vi "NI VeriStand - Start Single Waveform (CDB).vi"(8 "error in (no error)":errorcluster, 10 "t0":timestamp, 11 "Single Waveform Write Session (CDB) in":refnum<class "Single Waveform Write (CDB).lvclass">) -> (0 "error out":errorcluster, 3 "Single Waveform Write Session (CDB) out":refnum<class "Single Waveform Write (CDB).lvclass">)   [LabVIEW 2020, in "NI_VS Custom Device Waveform API.lvlib" / "Single Waveform Write (CDB).lvclass"]
doc: "Sets the start time (t0) for the waveform data you want to write with the Write Waveform(s) VI. NI VeriStand considers all data the custom device writes to a waveform be continuous unless this VI executes again with a different start time."
uses:
  Single Waveform Write (CDB).lvclass
  D:/p4/penguin/lvaddon/Veristand/master/src/LabVIEW/vilib/NI VeriStand/Custom Device Waveform API/Waveform Session.lvclass
  Waveform Session.lvclass/Waveform Session.ctl
  Single Waveform Write (CDB).lvclass/Single Waveform Write (CDB).ctl
  Internal Comm Classes/WPL Comm/WPL Comm.lvclass/WPL Comm.ctl
  Internal Comm Classes/WPL Comm/Set t0 on Variant.vi
  Internal Comm Classes/WPL Comm/Send WPL Command.vi
  Internal Comm Classes/WPL Comm/Convert Q Error to Shutdown Error.vi
  Internal Comm Classes/WPL Comm/WPL Comm (1D CDB)/WPL Comm (1D CDB).lvclass
  D:/p4/penguin/lvaddon/Veristand/master/src/LabVIEW/vilib/NI VeriStand/Custom Device Waveform API/Internal Comm Classes/WPL Comm/WPL Comm.lvclass
  <vilib>/Utility/error.llb/Error Cluster From Error Code.vi
  Internal Comm Classes/WPL Comm/WPL Comm.lvclass
  Waveform Session.lvclass
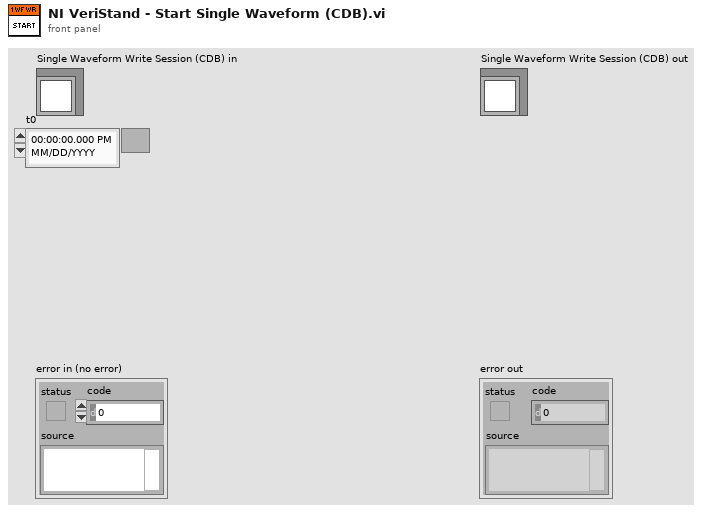
[diagram p1: front panel]
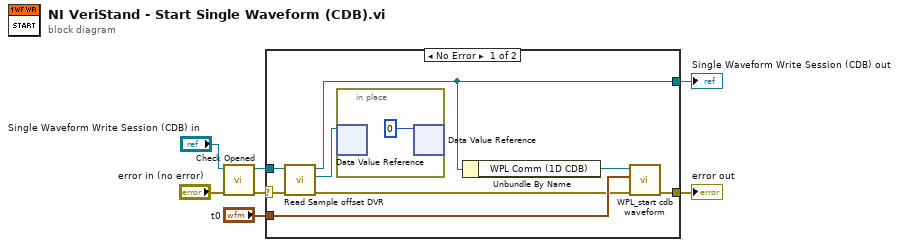
[diagram p0: block diagram]
diagram:
  n1 = call "Check Opened.vi"("error in (no error)"="error in (no error)", "Waveform Session in"="Single Waveform Write Session (CDB) in") -> ("error out"=w2:errorcluster, "Waveform Session out"=w1:refnum<class "Single Waveform Write (CDB).lvclass">)  [unwired: 8 in]
  n2 = case shown="No Error" w2 {
    selector: w2 -> [w8 w17]
    tunnel: [w13 w17] -> w7
    tunnel: [w9 w16] -> w6
    tunnel: w1 -> [w10 w16]
    tunnel: "t0" -> [w12 _]
    frame No Error {
      n3 = call "Read Sample offset DVR.vi"("Waveform Session in"=w10) -> ("Sample offset"=w11:refnum<data-value>, "Waveform Session out"=w9:refnum<class "Single Waveform Write (CDB).lvclass">)  [unwired: 9 in]
      n4 = in-place {
        n5 = in-place-dvr #1(w11) -> ()  [unwired: 2 out]
        n6 = in-place-dvr #1(u64 0 ("data value")) -> ()  [unwired: 2 out]
      }
      n7 = Unbundle By Name(w9) -> ("WPL Comm (1D CDB)"=w14:refnum<class "WPL Comm (1D CDB).lvclass">)
      n8 = call "WPL_start cdb waveform.vi"("error in (no error)"=w8, "t0"=w12, "WPL Comm in"=w14) -> ("error out"=w13:errorcluster)  [unwired: 8 in]
    }
    frame Error {
    }
  }
  "error out" <- w7
  "Single Waveform Write Session (CDB) out" <- w6
